vi "setUp.vi"(8 "error in (no error)":errorcluster, 11 "reference in":refnum<class "SLSC 12201 System Tests.lvclass">) -> (0 "error out":errorcluster, 3 "reference out":refnum<class "SLSC 12201 System Tests.lvclass">)   [LabVIEW 2017, in "SLSC 12201 System Tests.lvclass"]
doc: "setUp runs prior to the test method during test execution. Use this method to initialize any object data required by your tests."
uses:
  SLSC 12201 System Tests.lvclass
  <vilib>/addons/_JKI Toolkits/VI Tester/TestCase.llb/TestCase.lvclass
  C:/Program Files (x86)/National Instruments/LabVIEW 2019/vi.lib/addons/_JKI Toolkits/VI Tester/TestCase.llb/TestCase.lvclass
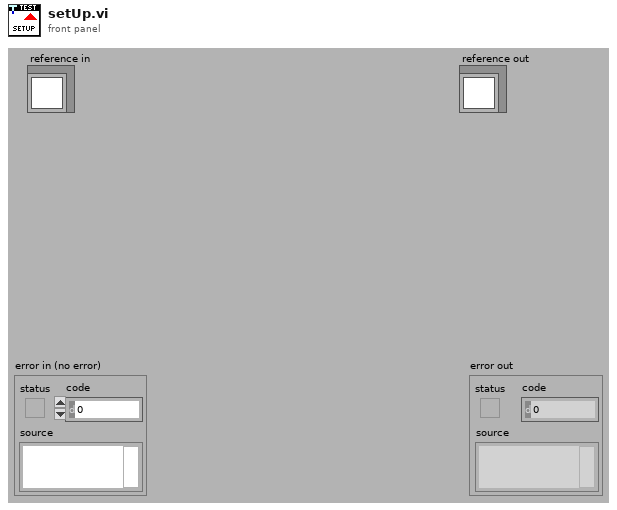
[diagram p1: front panel]
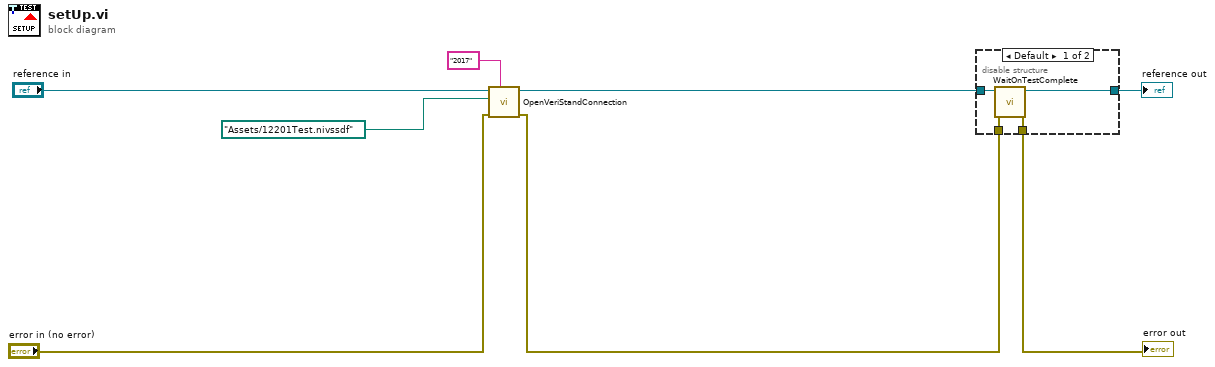
[diagram p0: block diagram]
diagram:
  n1 = call-dynamic "OpenVeriStandConnection.vi"("Minimum VeriStand Version (2015)"="2017", "error in (no error)"="error in (no error)", "System Definition File"=path "Assets/12201Test.nivssdf", "VeriStand Test Case in"="reference in") -> ("error out"=w3:errorcluster, "VeriStand Test Case out"=w5:refnum<class "SLSC 12201 System Tests.lvclass">)  [unwired: 5 in, 1 out]
  n2 = disable-structure shown="Default" {
    disable-tunnel: w3 -> [w12 w13]
    disable-tunnel: [w11 w13] -> w8
    disable-tunnel: [w10 w14] -> w6
    disable-tunnel: w5 -> [w9 w14]
    frame condition #0 (active) {
      n3 = call <vilib>:"WaitOnTestComplete.vi"("error in (no error)"=w12, "TestCase in"=w9) -> ("error out"=w11:errorcluster, "TestCase out"=w10:refnum<class "SLSC 12201 System Tests.lvclass">)  [unwired: 8 in]
    }
    frame condition #1 {
    }
  }
  "error out" <- w8
  "reference out" <- w6
